vi "参考-txt文本读写.vi"() -> ()   [LabVIEW 2021]
doc: "本范例演示“写入文本文件”和“读取文本文件”函数各种不同选项的用法。"
panel:
  out "读取文本（多行）":string[](array[string])
  in  "读取计数（多行）":i32=-1
  out "读取文本":string="\n"
  in  "写入文本":string="文本文件第一行。\n文本文件第二行。\n文本文件第三行。"
  in  "操作":u16(ring) items=["输入文件路径", "输入文件引用句柄", "取消勾选“转换EOL”", "“读取行”设为单行", "“读取行”设为多行"]
  # "概述：演示使用写入文本文件函数将数据写入文本文件，并通过读取文本文件函数从该文本文件中读取数据。\n操作步骤：\n1.将操作设置为“写入文本文件”函数和“读取文本文件”函数的某种特定用例。\n2.运行VI。以下“写入”值将被写入文件，然后再通过读取该文件重新加载并显示在“读取”值中。\n3.完成后删除文本文件（位于[LabVIEW Data]\\Example Write Read Text File.txt）。"
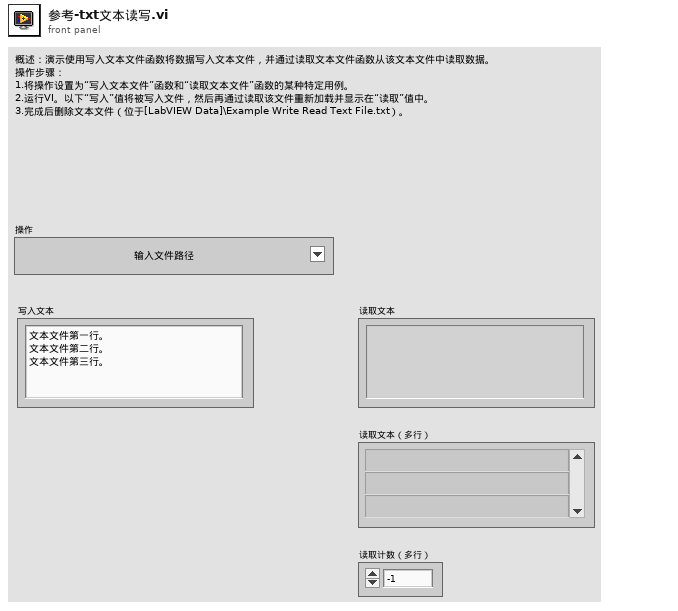
[diagram p1: front panel]
types:
  T1 = enum16{"open", "replace", "create", "open or create", "replace or create", "replace or create with confirmation"}
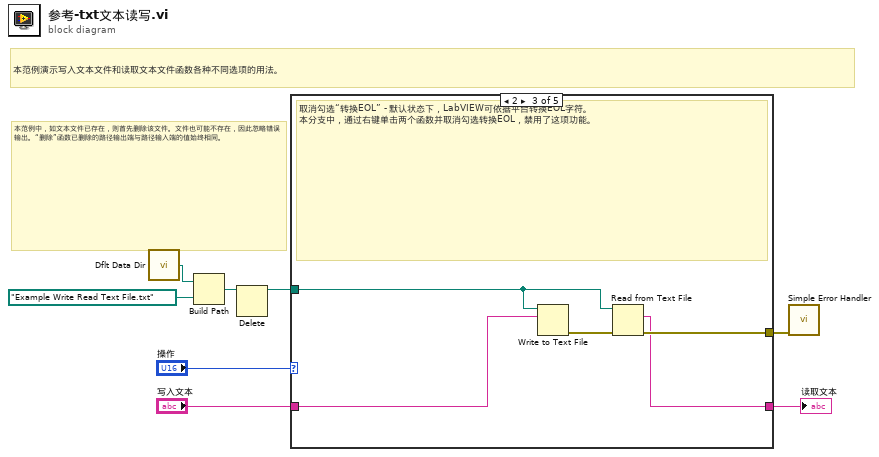
[diagram p0: block diagram]
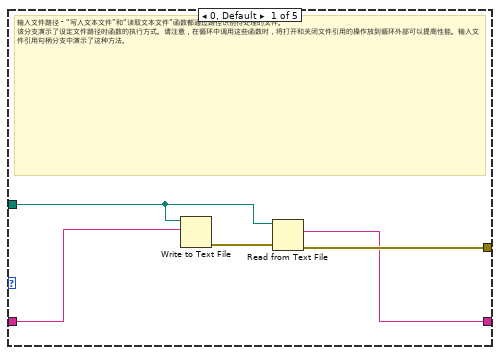
[diagram p2: hidden frame]
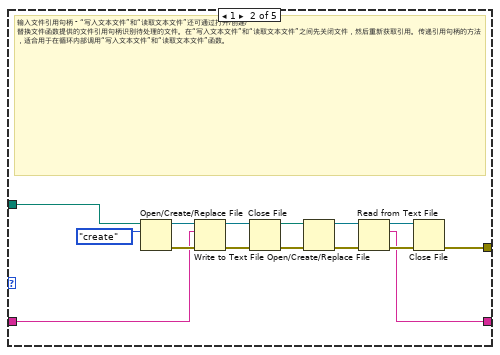
[diagram p3: hidden frame]
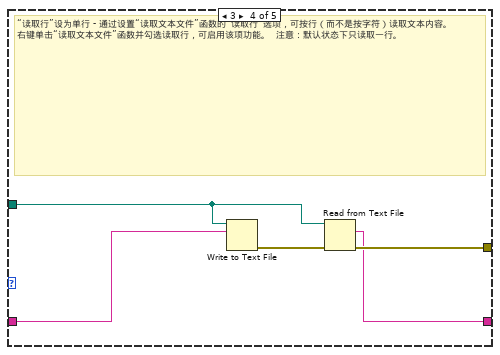
[diagram p4: hidden frame]
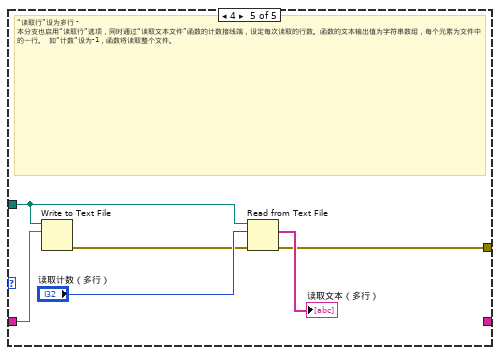
[diagram p5: hidden frame]
diagram:
  # "本范例演示写入文本文件和读取文本文件函数各种不同选项的用法。"
  # "本范例中，如文本文件已存在，则首先删除该文件。文件也可能不存在，因此忽略错误输出。“删除”函数已删除的路径输出端与路径输入端的值始终相同。"
  n1 = call <vilib>:"Dflt Data Dir.vi"() -> ("App:Default Data Directory"=w6:path)
  n2 = Build Path(base path=w6, name or relative path=path "Example Write Read Text File.txt" ("default name")) -> (appended path=w4:path)
  n3 = Delete(path (use dialog)=w4) -> (deleted path=w3:path)  [unwired: 4 in, 2 out]
  n4 = case shown="2" "操作" {
    tunnel: [w12 w23 w32 w37 w41] -> w1
    tunnel: "写入文本" -> [w11 w16 w31 w36 w40]
    tunnel: [w10 w15 w30 w35 _] -> w7
    tunnel: w3 -> [w9 w14 w29 w34 w39]
    frame 0, Default {
      # "输入文件路径 - “写入文本文件”和“读取文本文件”函数都通过路径识别待处理的文件。  该分支演示了设定文件路径时函数的执行方式。请注意，在循环中调用这些函数时，将打开和关闭文件引用的操作放到循环外部可以提高性能。输入文件引用句柄分支中演示了这种方法。"
      n5 = Write to Text File(file (use dialog)=w9, text=w11) -> (error out=w13:errorcluster)  [unwired: 2 in, 2 out]
      n6 = Read from Text File(file (use dialog)=w9, error in=w13) -> (text=w10:string, error out=w12:errorcluster)  [unwired: 2 in, 2 out]
    }
    frame 1 {
      # "输入文件引用句柄 - “写入文本文件”和“读取文本文件”还可通过打开/创建/替换文件函数提供的文件引用句柄识别待处理的文件。在“写入文本文件”和“读取文本文件”之间先关闭文件，然后重新获取引用。传递引用句柄的方法，适合用于在循环内部调用“写入文本文件”和“读取文本文件”函数。"
      n7 = Open/Create/Replace File(file path (use dialog)=w14, operation (0:open)=T1."create") -> (refnum out=w26:refnum<file>, error out=w28:errorcluster)  [unwired: 4 in, 1 out]
      n8 = Write to Text File(file (use dialog)=w26, text=w16, error in=w28) -> (refnum out=w22:refnum<file>, error out=w18:errorcluster)  [unwired: 1 in, 1 out]
      n9 = Close File(refnum=w22, error in=w18) -> (path=w21:path, error out=w20:errorcluster)
      n10 = Open/Create/Replace File(file path (use dialog)=w21, error in=w20) -> (refnum out=w19:refnum<file>, error out=w17:errorcluster)  [unwired: 4 in, 1 out]
      n11 = Read from Text File(file (use dialog)=w19, error in=w17) -> (refnum out=w25:refnum<file>, text=w15:string, error out=w24:errorcluster)  [unwired: 2 in, 1 out]
      n12 = Close File(refnum=w25, error in=w24) -> (error out=w23:errorcluster)  [unwired: 1 out]
    }
    frame 2 {
      # "取消勾选“转换EOL” - 默认状态下，LabVIEW可依据平台转换EOL字符。  本分支中，通过右键单击两个函数并取消勾选转换EOL，禁用了这项功能。"
      n13 = Write to Text File(file (use dialog)=w29, text=w31) -> (error out=w33:errorcluster)  [unwired: 2 in, 2 out]
      n14 = Read from Text File(file (use dialog)=w29, error in=w33) -> (text=w30:string, error out=w32:errorcluster)  [unwired: 2 in, 2 out]
    }
    frame 3 {
      # "“读取行”设为单行 - 通过设置“读取文本文件”函数的“读取行”选项，可按行（而不是按字符）读取文本内容。  右键单击“读取文本文件”函数并勾选读取行，可启用该项功能。  注意：默认状态下只读取一行。"
      n15 = Write to Text File(file (use dialog)=w34, text=w36) -> (error out=w38:errorcluster)  [unwired: 2 in, 2 out]
      n16 = Read from Text File(file (use dialog)=w34, error in=w38) -> (text=w35:string, error out=w37:errorcluster)  [unwired: 2 in, 2 out]
    }
    frame 4 {
      # "“读取行”设为多行 -  本分支也启用“读取行”选项，同时通过“读取文本文件”函数的计数接线端，设定每次读取的行数。函数的文本输出值为字符串数组，每个元素为文件中的一行。  如“计数”设为-1，函数将读取整个文件。"
      n17 = Write to Text File(file (use dialog)=w39, text=w40) -> (error out=w42:errorcluster)  [unwired: 2 in, 2 out]
      n18 = Read from Text File(file (use dialog)=w39, count="读取计数（多行）", error in=w42) -> (text=→"读取文本（多行）":string[], error out=w41:errorcluster)  [unwired: 1 in, 2 out]
    }
  }
  "读取文本" <- w7
  n19 = call <vilib>:"Simple Error Handler.vi"("error in (no error)"=w1) -> ()  [unwired: 4 in, 5 out]
